vi "UHR-Fleezers Control (host) - 11.8.vi"() -> ()   [LabVIEW 2014] (continued)
                    tunnel: w545 -> [w549 w564]
                    tunnel: [w548 w563] -> w543
                    tunnel: w542 -> [_ w559]
                    frame False {
                      n310 = local read "Fish"() -> (w548:bool)
                      n311 = case shown="False" w548 {
                        tunnel: w549 -> [w550 _]
                        frame False {
                          n312 = property on="BD 1 Frequency 1 (MHz)" class="DigNum (strict)"("Val(Sgnl)"=w550) -> ()  [unwired: 2 in, 2 out]
                        }
                        frame True {
                        }
                      }
                    }
                    frame True {
                      w563 = FALSE ("Fish for Tether")
                      n313 = call <vilib>:"Beep.vi"() -> ()  [unwired: 3 in, 9 out]
                      n314 = Number To Decimal String(number=w559, width (-)=i16 1) -> (decimal integer string=w557:string)
                      n315 = Concatenate Strings("Formed tether in ", w557, " attempt(s)." ("string")) -> (w554:string)
                      n316 = local read "Messages"() -> (w561:string)
                      n317 = local write "Fish"(w563) -> ()
                      n318 = call "Update messages.vi"("Message to add"=w554, "Old message string"=w561) -> ("New message string"=w560:string)
                      n319 = local write "Messages"(w560) -> ()
                      n320 = Get Date/Time In Seconds() -> (seconds since 1Jan1904=→"Time tether formed":timestamp)
                      n321 = local read "Flow ON\nduring cal?"() -> (w551:bool)
                      n322 = property on="Sample Channel\nFlow" class="Bool (strict)"("Val(Sgnl)"=w551) -> (error out=w552:errorcluster)  [unwired: 2 in, 1 out]
                      n323 = case shown="\"8\"" "Then..." {
                        selector: "Then..." -> [_ w567 _ _]
                        tunnel: w564 -> [w566 _ _ _]
                        tunnel: w552 -> [_ _ _ _]
                        frame "1", Default {
                          n324 = property on="BD 1 Frequency 1 (MHz)" class="DigNum (strict)"("Val(Sgnl)"=w566) -> ()  [unwired: 2 in, 2 out]
                        }
                        frame "2", "3", "4", "5", "6" {
                          n325 = flat-sequence {
                            tunnel: w567 -> [w569]
                            frame #0 {
                              n326 = property on="Trap D (MHz)" class="DigNum (strict)"("Val(Sgnl)"="Move to D 1 (MHz)") -> ()  [unwired: 2 in, 2 out]
                            }
                            frame #1 {
                              n327 = case shown="\"2\", Default" w569 {
                                selector: w569 -> [w572 w582 _]
                                frame "3", "4" {
                                n328 = flat-sequence {
                                tunnel: w572 -> [w573]
                                tunnel: [w573] -> w570
                                tunnel: [w575] -> w571
                                tunnel: w570 -> [w575]
                                tunnel: w571 -> [w579]
                                frame #0 {
                                n329 = property on="Green Laser ON/Interlacing" class="Bool (strict)"("Val(Sgnl)"=TRUE ("Value (Signaling)")) -> ()  [unwired: 2 in, 2 out]
                                }
                                frame #1 {
                                n330 = Multiply(x="Wait Before Save (s)", y=u32 1000 ("x")) -> (x*y=w577:u32)
                                n331 = Wait (ms)(milliseconds to wait=w577) -> ()  [unwired: 1 out]
                                }
                                frame #2 {
                                n332 = property on="Start Saving" class="Bool (strict)"("Value"=TRUE ("Start Saving")) -> ()  [unwired: 2 in, 2 out]
                                n333 = case shown="\"4\"" w579 {
                                frame Default {
                                }
                                frame "4" {
                                n334 = property on="Fl. Triggered..." class="Bool (strict)"("Val(Sgnl)"=TRUE ("Value (Signaling)")) -> ()  [unwired: 2 in, 2 out]
                                }
                                }
                                }
                                }
                                }
                                frame "5", "6" {
                                n335 = stacked-sequence {
                                tunnel: w582 -> [_ _ _ _ _ _ w594]
                                frame #0 {
                                n336 = Replace Array Subset(array=u32[] [0] ("Index Values"), new element="Raster Set\nUpon Tether", index=0) -> (w583:u32[])
                                n337 = property on="Saved AOD Raster Scan Parameter Sets" class="Arr (strict)"("Index Values"=w583) -> ()  [unwired: 2 in, 2 out]
                                }
                                frame #1 {
                                n338 = Wait (ms)(milliseconds to wait=u32 500) -> ()  [unwired: 1 out]
                                }
                                frame #2 {
                                n339 = property on="Load parameters" class="Bool (strict)"("Val(Sgnl)"=TRUE ("Value (Signaling)")) -> ()  [unwired: 2 in, 2 out]
                                n340 = case shown="True" "Green ON during\nraster?" {
                                frame False {
                                }
                                frame True {
                                n341 = property on="Green Laser ON/Interlacing" class="Bool (strict)"("Val(Sgnl)"=TRUE ("Value (Signaling)")) -> ()  [unwired: 2 in, 2 out]
                                }
                                }
                                }
                                frame #3 {
                                n342 = Wait (ms)(milliseconds to wait=u32 500) -> ()  [unwired: 1 out]
                                }
                                frame #4 {
                                n343 = property on="Trap Raster Scan" class="Bool (strict)"("Val(Sgnl)"=TRUE ("Value (Signaling)")) -> ()  [unwired: 2 in, 2 out]
                                }
                                frame #5 {
                                n344 = Wait (ms)(milliseconds to wait=u32 2000) -> ()  [unwired: 1 out]
                                }
                                frame #6 {
                                n345 = flat-sequence {
                                tunnel: w594 -> [w601]
                                frame #0 {
                                n346 = while {
                                stop <- w597 stop-if-true
                                n347 = local read "Raster Scanning..."() -> (w596:bool)
                                n348 = local read "Saving..."() -> (w599:bool)
                                n349 = Wait (ms)(milliseconds to wait=u32 100) -> ()  [unwired: 1 out]
                                n350 = Not(x=w599) -> (.not. x?=w598:bool)
                                n351 = Not(x=w596) -> (.not. x?=w595:bool)
                                n352 = And(x=w598, y=w595) -> (x .and. y?=w597:bool)
                                }
                                }
                                frame #1 {
                                n353 = local read "Tether"() -> (w602:bool)
                                n354 = case shown="True" w602 {
                                tunnel: w601 -> [_ w604]
                                frame False {
                                n355 = property on="Fish" class="Bool (strict)"("Val(Sgnl)"="Fish again after \nraster break?") -> ()  [unwired: 2 in, 2 out]
                                }
                                frame True {
                                n356 = stacked-sequence {
                                tunnel: w604 -> [_ w608 _ _ _ _ _ _]
                                frame #0 {
                                n357 = property on="Trap D (MHz)" class="DigNum (strict)"("Val(Sgnl)"="Move to D 2 (MHz)") -> ()  [unwired: 2 in, 2 out]
                                n358 = case shown="True" "Flow ON after\ntether testing?" {
                                frame False {
                                }
                                frame True {
                                n359 = property on="Sample Channel\nFlow" class="Bool (strict)"("Val(Sgnl)"=TRUE ("Value (Signaling)")) -> ()  [unwired: 2 in, 2 out]
                                }
                                }
                                }
                                frame #1 {
                                n360 = flat-sequence {
                                tunnel: w608 -> [w609]
                                frame #0 {
                                n361 = case shown="\"6\"" w609 {
                                frame Default {
                                }
                                frame "6" {
                                n362 = flat-sequence {
                                frame #0 {
                                n363 = Wait (ms)(milliseconds to wait=u32 500) -> ()  [unwired: 1 out]
                                }
                                frame #1 {
                                n364 = property on="Green Laser ON/Interlacing" class="Bool (strict)"("Val(Sgnl)"=TRUE ("Green Laser ON/Interlacing")) -> ()  [unwired: 2 in, 2 out]
                                }
                                }
                                }
                                }
                                }
                                frame #1 {
                                n365 = case shown="True" "Save at end (5, 6)" {
                                selector: "Save at end (5, 6)" -> [_ w613]
                                frame False {
                                }
                                frame True {
                                n366 = flat-sequence {
                                tunnel: w613 -> [w615]
                                frame #0 {
                                n367 = Wait (ms)(milliseconds to wait=u32 500) -> ()  [unwired: 1 out]
                                }
                                frame #1 {
                                n368 = local write "Start Saving"(w615) -> ()
                                }
                                }
                                }
                                }
                                }
                                }
                                }
                                frame #2 {
                                n369 = local read "Bead Sep. Int. Time (s)"() -> (w618:dbl)
                                n370 = Multiply(x=w618, y=1000.0) -> (x*y=w617:dbl)
                                n371 = Wait (ms)(milliseconds to wait=w617) -> ()  [unwired: 1 out]
                                }
                                frame #3 {
                                n372 = property on="Remove Offset" class="Bool (strict)"("Val(Sgnl)"=TRUE ("Value (Signaling)")) -> ()  [unwired: 2 in, 2 out]
                                }
                                frame #4 {
                                n373 = property on="Read FX file" class="Bool (strict)"("Val(Sgnl)"=TRUE ("Value (Signaling)")) -> ()  [unwired: 2 in, 2 out]
                                }
                                frame #5 {
                                n374 = Wait (ms)(milliseconds to wait=u32 300) -> ()  [unwired: 1 out]
                                }
                                frame #6 {
                                n375 = local read "Bad fit error"() -> (w627:dbl)
                                n376 = local read "Fit offset"() -> (w630:dbl)
                                n377 = Greater Or Equal?(x=w627, y="Bad fit thresh") -> (x >= y?=→"Bad fit":bool)
                                n378 = Greater Or Equal?(x=w630, y="Fit offset thresh") -> (x >= y?=→"Multiple tether":bool)
                                n379 = local read "Hyst. error"() -> (w624:dbl)
                                n380 = Greater Or Equal?(x=w624, y="Hysteresis thresh") -> (x >= y?=→"Hysteresis":bool)
                                }
                                frame #7 {
                                w635 = 0
                                n381 = local read "Bad fit error"() -> (w637:dbl)
                                n382 = local read "Hyst. error"() -> (w636:dbl)
                                n383 = local read "Fit offset"() -> (w638:dbl)
                                n384 = local read "Multiple tether"() -> (w644:bool)
                                n385 = local read "Hysteresis"() -> (w642:bool)
                                n386 = local read "Bad fit"() -> (w643:bool)
                                n387 = Not(x=w642) -> (.not. x?=w634:bool)
                                n388 = Not(x=w643) -> (.not. x?=w640:bool)
                                n389 = Greater?(x=w638, y=w635) -> (0:w633:bool)
                                n390 = Greater?(x=w637, y=w635) -> (0:w632:bool)
                                n391 = Greater?(x=w636, y=w635) -> (0:w631:bool)
                                n392 = Not(x=w644) -> (.not. x?=w641:bool)
                                n393 = Compound Arithmetic op=AND(w641, w640, w634, w633, w632, w631) -> (w639:bool)
                                "Good tether" <- w639
                                n394 = case shown="True" w639 {
                                frame False {
                                }
                                frame True {
                                n395 = call <vilib>:"Beep.vi"("use system alert? (T)"=FALSE, "duration (msec)"=u32 200, "frequency (Hz)"=u32 2000) -> ()  [unwired: 9 in]
                                }
                                }
                                }
                                }
                                }
                                }
                                }
                                }
                                }
                                }
                                }
                                frame "2", Default {
                                }
                              }
                            }
                            frame #2 {
                              n396 = local read "Multiple tether"() -> (w650:bool)
                              n397 = And(x="Break multiple", y=w650) -> (x .and. y?=w648:bool)
                              n398 = case shown="True" w648 {
                                frame False {
                                }
                                frame True {
                                n399 = stacked-sequence {
                                frame #0 {
                                n400 = property on="Trap D (MHz)" class="DigNum (strict)"("Val(Sgnl)"="Trap D to \nbreak (MHz)") -> ()  [unwired: 2 in, 2 out]
                                }
                                frame #1 {
                                n401 = case shown="True" "Fish after\nmultiple break" {
                                frame False {
                                }
                                frame True {
                                n402 = while {
                                stop <- w655 stop-if-true
                                n403 = local read "Multiple tether"() -> (w657:bool)
                                n404 = local read "Fish"() -> (w654:bool)
                                n405 = local read "Stop All"() -> (w653:bool)
                                n406 = Wait (ms)(milliseconds to wait=u32 100) -> ()  [unwired: 1 out]
                                n407 = Not(x=w657) -> (.not. x?=w656:bool)
                                n408 = Compound Arithmetic op=OR(w653, w656, w654) -> (w655:bool)
                                }
                                }
                                }
                                }
                                frame #2 {
                                n409 = local read "Fish after\nmultiple break"() -> (w662:bool)
                                n410 = local read "Stage Moving"() -> (w661:bool)
                                n411 = Not(x=w661) -> (.not. x?=w659:bool)
                                n412 = And(x=w662, y=w659) -> (x .and. y?=w660:bool)
                                n413 = property on="Fish" class="Bool (strict)"("Val(Sgnl)"=w660) -> ()  [unwired: 2 in, 2 out]
                                }
                                }
                                }
                              }
                            }
                            frame #3 {
                              n414 = local read "Bad fit"() -> (w664:bool)
                              n415 = And(x="Break bad fit", y=w664) -> (x .and. y?=w663:bool)
                              n416 = case shown="True" w663 {
                                frame False {
                                }
                                frame True {
                                n417 = stacked-sequence {
                                frame #0 {
                                n418 = local read "Trap D to \nbreak (MHz)"() -> (w666:dbl)
                                n419 = property on="Trap D (MHz)" class="DigNum (strict)"("Val(Sgnl)"=w666) -> ()  [unwired: 2 in, 2 out]
                                }
                                frame #1 {
                                n420 = case shown="True" "Fish after\nbad fit break?" {
                                frame False {
                                }
                                frame True {
                                n421 = while {
                                stop <- w670 stop-if-true
                                n422 = local read "Stop All"() -> (w668:bool)
                                n423 = local read "Bad fit"() -> (w669:bool)
                                n424 = local read "Fish"() -> (w671:bool)
                                n425 = Not(x=w669) -> (.not. x?=w672:bool)
                                n426 = Wait (ms)(milliseconds to wait=u32 100) -> ()  [unwired: 1 out]
                                n427 = Compound Arithmetic op=OR(w668, w672, w671) -> (w670:bool)
                                }
                                }
                                }
                                }
                                frame #2 {
                                n428 = local read "Fish after\nbad fit break?"() -> (w674:bool)
                                n429 = local read "Stage Moving"() -> (w677:bool)
                                n430 = Not(x=w677) -> (.not. x?=w676:bool)
                                n431 = And(x=w674, y=w676) -> (x .and. y?=w675:bool)
                                n432 = property on="Fish" class="Bool (strict)"("Val(Sgnl)"=w675) -> ()  [unwired: 2 in, 2 out]
                                }
                                }
                                }
                              }
                            }
                            frame #4 {
                              n433 = local read "Hysteresis"() -> (w679:bool)
                              n434 = And(x="Break hyst", y=w679) -> (x .and. y?=w678:bool)
                              n435 = case shown="True" w678 {
                                frame False {
                                }
                                frame True {
                                n436 = stacked-sequence {
                                frame #0 {
                                n437 = local read "Trap D to \nbreak (MHz)"() -> (w681:dbl)
                                n438 = property on="Trap D (MHz)" class="DigNum (strict)"("Val(Sgnl)"=w681) -> ()  [unwired: 2 in, 2 out]
                                }
                                frame #1 {
                                n439 = case shown="True" "Fish ater hyst?" {
                                frame False {
                                }
                                frame True {
                                n440 = while {
                                stop <- w687 stop-if-true
                                n441 = local read "Hysteresis"() -> (w686:bool)
                                n442 = local read "Stop All"() -> (w683:bool)
                                n443 = local read "Fish"() -> (w684:bool)
                                n444 = Wait (ms)(milliseconds to wait=u32 100) -> ()  [unwired: 1 out]
                                n445 = Not(x=w686) -> (.not. x?=w685:bool)
                                n446 = Compound Arithmetic op=OR(w683, w685, w684) -> (w687:bool)
                                }
                                }
                                }
                                }
                                frame #2 {
                                n447 = local read "Fish ater hyst?"() -> (w692:bool)
                                n448 = local read "Stage Moving"() -> (w691:bool)
                                n449 = Not(x=w691) -> (.not. x?=w690:bool)
                                n450 = And(x=w692, y=w690) -> (x .and. y?=w689:bool)
                                n451 = property on="Fish" class="Bool (strict)"("Val(Sgnl)"=w689) -> ()  [unwired: 2 in, 2 out]
                                }
                                }
                                }
                              }
                            }
                            frame #5 {
                              n452 = local read "Good tether"() -> (w693:bool)
                              n453 = case shown="True" w693 {
                                frame False {
                                }
                                frame True {
                                n454 = case shown="\"1\"" "If good, then:" {
                                frame "0", Default {
                                }
                                frame "1" {
                                n455 = property on="Force FB Script" class="Bool (strict)"("Val(Sgnl)"=TRUE ("Value (Signaling)")) -> ()  [unwired: 2 in, 2 out]
                                }
                                }
                                }
                              }
                            }
                          }
                        }
                        frame "7" {
                          n456 = property on="Force FB Script" class="Bool (strict)"("Val(Sgnl)"=TRUE ("Value (Signaling)")) -> ()  [unwired: 2 in, 2 out]
                        }
                        frame "8" {
                          n457 = property on="Fixed Traps Script" class="Bool (strict)"("Val(Sgnl)"=TRUE ("Value (Signaling)")) -> ()  [unwired: 2 in, 2 out]
                        }
                      }
                      "Tether" <- "Tether Alarm?"
                    }
                  }
                }
                frame #2 {
                  n458 = local read "Oscillate Set 1"() -> (w703:bool)
                  n459 = local read "Stop All"() -> (w701:bool)
                  n460 = Or(x=w703, y=w698) -> (x .or. y?=w700:bool)
                  n461 = Not(x=w700) -> (.not. x?=w702:bool)
                  n462 = Compound Arithmetic op=OR(w701, w702) -> (w699:bool)
                }
              }
              n463 = node-c288() -> ()  [unwired: 2 out]
            }
            n464 = node-c288(w457) -> ()  [unwired: 1 out]
          }
        }
      }
      event "Fl. Triggered...": Value Change {
        n465 = event-data() -> ()  [unwired: 7 out]
        n466 = case shown="True" "Fl. Triggered..." {
          frame False {
          }
          frame True {
            n467 = node-c288() -> (w714:T21)  [unwired: 4 out]
            n468 = timed-loop {
              timing: w714 -> [_]
              timing-out: [_] -> w713
              tunnel: "Action" -> [w722]
              shift-right: [w719] -> _
              shift-left: u8 255 -> [w721]
              shift-right: [w716] -> _
              shift-left: 255 -> [w718]
              stop <- w715 stop-if-true
              # "Reset confocal spot"
              n469 = node-c288() -> ()  [unwired: 2 out]
              n470 = flat-sequence {
                tunnel: w722 -> [w742]
                tunnel: w721 -> [w741]
                tunnel: [w740] -> w720
                tunnel: w718 -> [w727]
                tunnel: [w726] -> w717
                tunnel: [w1126] -> w715
                tunnel: w720 -> [w1125]
                tunnel: [w1125] -> w719
                tunnel: [w1124] -> w716
                tunnel: w717 -> [w1124]
                frame #0 {
                  n471 = local read "Delta Fl. 2"() -> (w739:dbl)
                  n472 = local read "Delta Fl. 1"() -> (w734:dbl)
                  n473 = Multiply(x="Fl. D Thresh. (kHz)", y=1000.0) -> (x*y=w729:dbl)
                  n474 = Select(t=w734, s="APD to Watch", f=w739) -> (s? t:f=w730:dbl)
                  n475 = Greater?(x=w730, y=w729) -> (0:w735:bool)
                  n476 = Or(x="Force Yank", y=w735) -> (x .or. y?=w733:bool)
                  n477 = And(x=w733, y="Yank when?") -> (x .and. y?=w731:bool)
                  n478 = case shown="False" w731 {
                    tunnel: w742 -> [w745 w948]
                    tunnel: w741 -> [w747 w944]
                    tunnel: [w747 w942] -> w740
                    tunnel: w730 -> [w753 _]
                    tunnel: w729 -> [w752 _]
                    tunnel: "Force Yank" -> [w750 _]
                    tunnel: w727 -> [w749 w941]
                    tunnel: [w748 w941] -> w726
                    frame False {
                      n479 = Negate(x=w752) -> (-x=w744:dbl)
                      n480 = local write "Fl. High"(TRUE ("Fl. High")) -> ()
                      n481 = Less?(x=w753, y=w744) -> (x < y?=w751:bool)
                      n482 = Or(x=w750, y=w751) -> (x .or. y?=w746:bool)
                      n483 = case shown="True" w746 {
                        tunnel: w749 -> [w754 w764]
                        tunnel: [w754 w763] -> w748
                        tunnel: w745 -> [_ w762]
                        frame False {
                        }
                        frame True {
                          n484 = flat-sequence {
                            tunnel: w764 -> [w770]
                            tunnel: w762 -> [w767]
                            tunnel: [w769] -> w761
                            tunnel: [w768] -> w760
                            tunnel: [w767] -> w759
                            tunnel: w758 -> [w766]
                            tunnel: [w766] -> w757
                            tunnel: w756 -> [w765]
                            tunnel: [w765] -> w755
                            tunnel: [w842] -> w763
                            tunnel: w761 -> [w842]
                            tunnel: w760 -> [w841]
                            tunnel: w759 -> [w840]
                            tunnel: w757 -> [w839]
                            tunnel: w755 -> [w838]
                            frame #0 {
                              n485 = call <vilib>:"Beep.vi"() -> ()  [unwired: 12 in]
                              n486 = local write "Waiting"(FALSE ("Waiting")) -> ()
                              n487 = Increment(x=w770) -> (x+1=w769:i32)
                              n488 = case shown="\"Yank\"" w767 {
                                tunnel: w769 -> [_ w775 _]
                                frame "Alarm", Default {
                                }
                                frame "Yank" {
                                n489 = flat-sequence {
                                tunnel: w775 -> [w778]
                                tunnel: [w777] -> w774
                                tunnel: [w776] -> w773
                                tunnel: w774 -> [w788]
                                tunnel: w773 -> [w789]
                                frame #0 {
                                n490 = local read "Yank Delay (s)"() -> (w781:dbl)
                                n491 = local read "N Array El"() -> (w776:u8)
                                n492 = Quotient & Remainder(x=w778, y=w776) -> (x-y*floor(x/y)=w777:i32)  [unwired: 1 out]
                                n493 = Multiply(x=w781, y=1000.0) -> (x*y=w779:dbl)
                                n494 = Wait (ms)(milliseconds to wait=w779) -> ()  [unwired: 1 out]
                                }
                                frame #1 {
                                n495 = local read "Yank to which?"() -> (w783:bool)
                                n496 = local read "Random Choice"() -> (w793:bool)
                                n497 = local read "Yank to Trap D (MHz)"() -> (w786:dbl[])
                                n498 = local read "Yank to SP"() -> (w787:dbl[])
                                n499 = Random Number (0-1)() -> (number: 0 to 1=w792:dbl)
                                n500 = Multiply(x=w789, y=w792) -> (x*y=w791:dbl)
                                n501 = Round Toward -Infinity(1:w791) -> (0:w790:dbl)
                                n502 = Select(t=w790, s=w793, f=w788) -> (s? t:f=w784:dbl)
                                n503 = Select(t=w786, s=w783, f=w787) -> (s? t:f=w785:dbl[])
                                n504 = Index Array(array=w785, index=w784) -> (element=w782:dbl)
                                n505 = case shown="False" w783 {
                                tunnel: w782 -> [w794 w822]
                                frame False {
                                n506 = flat-sequence {
                                tunnel: w794 -> [w795]
                                frame #0 {
                                n507 = property on="Trap Pos FB SP" class="DigNum (strict)"("Val(Sgnl)"=w795) -> ()  [unwired: 2 in, 2 out]
                                }
                                frame #1 {
                                n508 = Wait (ms)(milliseconds to wait=u32 700) -> ()  [unwired: 1 out]
                                }
                                frame #2 {
                                n509 = local read "Action (%)"() -> (w800:dbl)
                                n510 = Absolute Value(x=w800) -> (abs(x)=w799:dbl)
                                n511 = Greater?(x=w799, y=70.0) -> (0:w797:bool)
                                n512 = property on="Remove Action Offset" class="Bool (strict)"("Val(Sgnl)"=w797) -> ()  [unwired: 2 in, 2 out]
                                }
                                frame #3 {
                                n513 = for {
                                N: 4 -> [_]
                                n514 = flat-sequence {
                                frame #0 {
                                n515 = Wait (ms)(milliseconds to wait=u32 500) -> ()  [unwired: 1 out]
                                }
                                frame #1 {
                                n516 = local read "Action (%)"() -> (w806:dbl)
                                n517 = Absolute Value(x=w806) -> (abs(x)=w805:dbl)
                                n518 = Greater?(x=w805, y=70.0) -> (0:w803:bool)
                                n519 = property on="Remove Action Offset" class="Bool (strict)"("Val(Sgnl)"=w803) -> ()  [unwired: 2 in, 2 out]
                                }
                                }
                                }
                                }
                                frame #4 {
                                n520 = Wait (ms)(milliseconds to wait=u32 500) -> ()  [unwired: 1 out]
                                }
                                frame #5 {
                                n521 = local read "Mean"() -> (w814:dbl)
                                n522 = Greater?(x=w814, y=11.0) -> (0:w808:bool)
                                n523 = Not(x=w808) -> (.not. x?=w809:bool)
                                n524 = And(x=w809, y="Shift confocal") -> (x .and. y?=w811:bool)
                                n525 = And(x=w808, y="Shift confocal") -> (x .and. y?=w812:bool)
                                n526 = case shown="True" w812 {
                                frame False {
                                }
                                frame True {
                                n527 = local read "Confocal Y 2 (V)"() -> (w818:dbl)
                                n528 = local read "Confocal X 2 (V)"() -> (w817:dbl)
                                n529 = property on="AO1" class="Slide (strict)"("Val(Sgnl)"=w818) -> ()  [unwired: 2 in, 2 out]
                                n530 = property on="AO2" class="Slide (strict)"("Val(Sgnl)"=w817) -> ()  [unwired: 2 in, 2 out]
                                }
                                }
                                n531 = case shown="True" w811 {
                                frame False {
                                }
                                frame True {
                                n532 = local read "Confocal Y 1 (V)"() -> (w816:dbl)
                                n533 = local read "Confocal X 1 (V)"() -> (w815:dbl)
                                n534 = property on="AO1" class="Slide (strict)"("Val(Sgnl)"=w816) -> ()  [unwired: 2 in, 2 out]
                                n535 = property on="AO2" class="Slide (strict)"("Val(Sgnl)"=w815) -> ()  [unwired: 2 in, 2 out]
                                }
                                }
                                }
                                frame #6 {
                                n536 = Wait (ms)(milliseconds to wait=u32 1500) -> ()  [unwired: 1 out]
                                }
                                frame #7 {
                                n537 = property on="Rem fb disp offset" class="Bool (strict)"("Val(Sgnl)"=TRUE ("Value (Signaling)")) -> ()  [unwired: 2 in, 2 out]
                                n538 = property on="Remove Offset" class="Bool (strict)"("Val(Sgnl)"=TRUE ("Value (Signaling)")) -> ()  [unwired: 2 in, 2 out]
                                }
                                }
                                }
                                frame True {
                                n539 = flat-sequence {
                                tunnel: w822 -> [w823]
                                frame #0 {
                                n540 = property on="Trap D (MHz)" class="DigNum (strict)"("Val(Sgnl)"=w823) -> ()  [unwired: 2 in, 2 out]
                                }
                                frame #1 {
                                n541 = Wait (ms)(milliseconds to wait=u32 500) -> ()  [unwired: 1 out]
                                }
                                frame #2 {
                                n542 = local read "Shift confocal"() -> (w829:bool)
                                n543 = local read "Mean"() -> (w831:dbl)
                                n544 = Greater?(x=w831, y=11.0) -> (0:w828:bool)
                                n545 = Not(x=w828) -> (.not. x?=w827:bool)
                                n546 = And(x=w827, y=w829) -> (x .and. y?=w825:bool)
                                n547 = And(x=w828, y=w829) -> (x .and. y?=w826:bool)
                                n548 = case shown="True" w826 {
                                frame False {
                                }
                                frame True {
                                n549 = local read "Confocal Y 2 (V)"() -> (w835:dbl)
                                n550 = local read "Confocal X 2 (V)"() -> (w834:dbl)
                                n551 = property on="AO2" class="Slide (strict)"("Val(Sgnl)"=w834) -> ()  [unwired: 2 in, 2 out]
                                n552 = property on="AO1" class="Slide (strict)"("Val(Sgnl)"=w835) -> ()  [unwired: 2 in, 2 out]
                                }
                                }
                                n553 = case shown="True" w825 {
                                frame False {
                                }
                                frame True {
                                n554 = local read "Confocal X 1 (V)"() -> (w832:dbl)
                                n555 = local read "Confocal Y 1 (V)"() -> (w833:dbl)
                                n556 = property on="AO2" class="Slide (strict)"("Val(Sgnl)"=w832) -> ()  [unwired: 2 in, 2 out]
                                n557 = property on="AO1" class="Slide (strict)"("Val(Sgnl)"=w833) -> ()  [unwired: 2 in, 2 out]
                                }
                                }
                                }
                                }
                                }
                                }
                                }
                                }
                                }
                                frame "Image" {
                                n558 = property on="Confocal\nImage" class="Bool (strict)"("Val(Sgnl)"=TRUE ("Value (Signaling)")) -> ()  [unwired: 2 in, 2 out]
                                }
                              }
                              n559 = local write "Fl. High"(FALSE ("Fl. High")) -> ()
                              n560 = local read "Time (s)"() -> (w768:dbl)
                            }
                            frame #1 {
                              n561 = case shown="True" "Auto F Reset" {
                                tunnel: w841 -> [_ w846]
                                tunnel: w840 -> [_ w845]
                                tunnel: w839 -> [_ w844]
                                tunnel: w838 -> [_ w843]
                                frame False {
                                }
                                frame True {
                                n562 = node-c288() -> (w848:T21)  [unwired: 4 in]
                                n563 = timed-loop {
                                timing: w848 -> [_]
                                timing-out: [_] -> w847
                                tunnel: w846 -> [w853]
                                tunnel: w845 -> [w852]
                                tunnel: w844 -> [w851]
                                tunnel: w843 -> [w850]
                                stop <- w849 stop-if-true
                                n564 = node-c288() -> ()  [unwired: 1 in, 1 out]
                                n565 = local read "APD to Watch"() -> (w863:bool)
                                n566 = local read "Fl. D Thresh. (kHz)"() -> (w862:dbl)
                                n567 = local read "Delta Fl. 1"() -> (w864:dbl)
                                n568 = local read "Delta Fl. 2"() -> (w865:dbl)
                                n569 = local read "Fl. Triggered..."() -> (w856:bool)
                                n570 = local read "Stop All"() -> (w857:bool)
                                n571 = local read "Reset Force"() -> (w855:bool)
                                n572 = Multiply(x=w862, y=1000.0) -> (x*y=w860:dbl)
                                n573 = Not(x=w856) -> (.not. x?=w854:bool)
                                n574 = Select(t=w864, s=w863, f=w865) -> (s? t:f=w859:dbl)
                                n575 = Greater?(x=w859, y=w860) -> (0:w858:bool)
                                n576 = Compound Arithmetic op=OR(w858, w857, w854, w855) -> (w849:bool)
                                n577 = case shown="True" w849 {
                                tunnel: w853 -> [_ w869]
                                tunnel: w852 -> [_ w873]
                                tunnel: w851 -> [_ w872]
                                tunnel: w850 -> [_ w871]
                                frame False {
                                }
                                frame True {
                                n578 = case shown="\"Yank\"" w873 {
                                tunnel: w872 -> [_ w883]
                                tunnel: w871 -> [_ w881]
                                frame "Image", Default {
                                }
                                frame "Yank" {
                                n579 = flat-sequence {
                                tunnel: [w886] -> w884
                                tunnel: w883 -> [w886]
                                tunnel: [w885] -> w882
                                tunnel: w881 -> [w885]
                                tunnel: w884 -> [w892]
                                tunnel: w882 -> [w890]
                                frame #0 {
                                n580 = local read "Yank Delay (s)"() -> (w889:dbl)
                                n581 = Multiply(x=w889, y=1000.0) -> (x*y=w887:dbl)
                                n582 = Wait (ms)(milliseconds to wait=w887) -> ()  [unwired: 1 out]
                                }
                                frame #1 {
                                n583 = local read "Yank to which?"() -> (w891:bool)
                                n584 = case shown="False" w891 {
                                tunnel: w892 -> [_ w921]
                                tunnel: w890 -> [w893 _]
                                frame False {
                                n585 = flat-sequence {
                                tunnel: w893 -> [w894]
                                frame #0 {
                                n586 = property on="Trap Pos FB SP" class="DigNum (strict)"("Val(Sgnl)"=w894) -> ()  [unwired: 2 in, 2 out]
                                }
                                frame #1 {
                                n587 = Wait (ms)(milliseconds to wait=u32 700) -> ()  [unwired: 1 out]
                                }
                                frame #2 {
                                n588 = local read "Action (%)"() -> (w899:dbl)
                                n589 = Absolute Value(x=w899) -> (abs(x)=w898:dbl)
                                n590 = Greater?(x=w898, y=70.0) -> (0:w896:bool)
                                n591 = property on="Remove Action Offset" class="Bool (strict)"("Val(Sgnl)"=w896) -> ()  [unwired: 2 in, 2 out]
                                }
                                frame #3 {
                                n592 = for {
                                N: 4 -> [_]
                                n593 = flat-sequence {
                                frame #0 {
                                n594 = Wait (ms)(milliseconds to wait=u32 500) -> ()  [unwired: 1 out]
                                }
                                frame #1 {
                                n595 = local read "Action (%)"() -> (w905:dbl)
                                n596 = Absolute Value(x=w905) -> (abs(x)=w904:dbl)
                                n597 = Greater?(x=w904, y=70.0) -> (0:w902:bool)
                                n598 = property on="Remove Action Offset" class="Bool (strict)"("Val(Sgnl)"=w902) -> ()  [unwired: 2 in, 2 out]
                                }
                                }
                                }
                                }
                                frame #4 {
                                n599 = Wait (ms)(milliseconds to wait=u32 500) -> ()  [unwired: 1 out]
                                }
                                frame #5 {
                                n600 = local read "Shift confocal"() -> (w910:bool)
                                n601 = local read "Mean"() -> (w913:dbl)
                                n602 = Greater?(x=w913, y=11.0) -> (0:w909:bool)
                                n603 = Not(x=w909) -> (.not. x?=w908:bool)
                                n604 = And(x=w909, y=w910) -> (x .and. y?=w911:bool)
                                n605 = And(x=w908, y=w910) -> (x .and. y?=w907:bool)
                                n606 = case shown="True" w911 {
                                frame False {
                                }
                                frame True {
                                n607 = local read "Confocal X 2 (V)"() -> (w916:dbl)
                                n608 = local read "Confocal Y 2 (V)"() -> (w917:dbl)
                                n609 = property on="AO2" class="Slide (strict)"("Val(Sgnl)"=w916) -> ()  [unwired: 2 in, 2 out]
                                n610 = property on="AO1" class="Slide (strict)"("Val(Sgnl)"=w917) -> ()  [unwired: 2 in, 2 out]
                                }
                                }
                                n611 = case shown="True" w907 {
                                frame False {
                                }
                                frame True {
                                n612 = local read "Confocal Y 1 (V)"() -> (w915:dbl)
                                n613 = local read "Confocal X 1 (V)"() -> (w914:dbl)
                                n614 = property on="AO1" class="Slide (strict)"("Val(Sgnl)"=w915) -> ()  [unwired: 2 in, 2 out]
                                n615 = property on="AO2" class="Slide (strict)"("Val(Sgnl)"=w914) -> ()  [unwired: 2 in, 2 out]
                                }
                                }
                                }
                                frame #6 {
                                n616 = Wait (ms)(milliseconds to wait=u32 1500) -> ()  [unwired: 1 out]
                                }
                                frame #7 {
                                n617 = property on="Remove Offset" class="Bool (strict)"("Val(Sgnl)"=TRUE ("Value (Signaling)")) -> ()  [unwired: 2 in, 2 out]
                                n618 = property on="Rem fb disp offset" class="Bool (strict)"("Val(Sgnl)"=TRUE ("Value (Signaling)")) -> ()  [unwired: 2 in, 2 out]
                                }
                                }
                                }
                                frame True {
                                n619 = flat-sequence {
                                tunnel: w921 -> [w922]
                                frame #0 {
                                n620 = property on="Trap D (MHz)" class="DigNum (strict)"("Val(Sgnl)"=w922) -> ()  [unwired: 2 in, 2 out]
                                }
                                frame #1 {
                                n621 = Wait (ms)(milliseconds to wait=u32 500) -> ()  [unwired: 1 out]
                                }
                                frame #2 {
                                n622 = local read "Shift confocal"() -> (w928:bool)
                                n623 = local read "Mean"() -> (w929:dbl)
                                n624 = Greater?(x=w929, y=11.0) -> (0:w927:bool)
                                n625 = And(x=w927, y=w928) -> (x .and. y?=w925:bool)
                                n626 = Not(x=w927) -> (.not. x?=w926:bool)
                                n627 = And(x=w926, y=w928) -> (x .and. y?=w924:bool)
                                n628 = case shown="True" w925 {
                                frame False {
                                }
                                frame True {
                                n629 = local read "Confocal Y 2 (V)"() -> (w934:dbl)
                                n630 = local read "Confocal X 2 (V)"() -> (w933:dbl)
                                n631 = property on="AO1" class="Slide (strict)"("Val(Sgnl)"=w934) -> ()  [unwired: 2 in, 2 out]
                                n632 = property on="AO2" class="Slide (strict)"("Val(Sgnl)"=w933) -> ()  [unwired: 2 in, 2 out]
                                }
                                }
                                n633 = case shown="True" w924 {
                                frame False {
                                }
                                frame True {
                                n634 = local read "Confocal Y 1 (V)"() -> (w932:dbl)
                                n635 = local read "Confocal X 1 (V)"() -> (w931:dbl)
                                n636 = property on="AO2" class="Slide (strict)"("Val(Sgnl)"=w931) -> ()  [unwired: 2 in, 2 out]
                                n637 = property on="AO1" class="Slide (strict)"("Val(Sgnl)"=w932) -> ()  [unwired: 2 in, 2 out]
                                }
                                }
                                }
                                }
                                }
                                }
                                }
                                }
                                }
                                }
                                n638 = local read "Time (s)"() -> (w868:dbl)
                                n639 = Subtract(x=w869, y=w868) -> (x-y=w880:dbl)
                                n640 = Number To Decimal String(number=w880, width (-)=i16 0) -> (decimal integer string=w878:string)
                                n641 = Concatenate Strings(w878, " s fluorescence event") -> (w875:string)
                                n642 = local read "Messages"() -> (w876:string)
                                n643 = local write "Duration (s)"(w880) -> ()
                                n644 = call "Update messages.vi"("Message to add"=w875, "Old message string"=w876) -> ("New message string"=w874:string)
                                n645 = local write "Messages"(w874) -> ()
                                n646 = call <vilib>:"Beep.vi"() -> ()  [unwired: 12 in]
                                n647 = local write "Reset Force"(FALSE ("Force Reset")) -> ()
                                n648 = local write "Fl. High"(TRUE ("Fl. High")) -> ()
                                n649 = local write "Waiting"(TRUE ("Waiting")) -> ()
                                }
                                }
                                n650 = node-c288() -> ()  [unwired: 1 in, 1 out]
                                }
                                n651 = node-c288(w847) -> ()  [unwired: 1 out]
                                }
                              }
                            }
                          }
                          n652 = local read "Trap Pos FB SP"() -> (w756:fxp<+/-,16,1>)
                          n653 = local read "Trap D (MHz)"() -> (w758:dbl)
                        }
                      }
                    }
                    frame True {
                      n654 = flat-sequence {
                        tunnel: w945 -> [w955]
                        tunnel: [w955] -> w949
                        tunnel: w948 -> [w954]
                        tunnel: [w954] -> w947
                        tunnel: [w953] -> w946
                        tunnel: w944 -> [w952]
                        tunnel: [w951] -> w943
                        tunnel: w940 -> [w950]
                        tunnel: [w950] -> w939
                        tunnel: w949 -> [w1027]
                        tunnel: w947 -> [w1026]
                        tunnel: w946 -> [w1025]
                        tunnel: w943 -> [w1024]
                        tunnel: w939 -> [w1023]
                        tunnel: [w1024] -> w942
                        frame #0 {
                          n655 = call <vilib>:"Beep.vi"() -> ()  [unwired: 3 in, 9 out]
                          n656 = local write "Waiting"(FALSE ("Waiting")) -> ()
                          n657 = Increment(x=w952) -> (x+1=w951:u8)
                          n658 = case shown="\"Image\"" w954 {
                            tunnel: w951 -> [_ _ w961 _]
                            frame "Image" {
                              n659 = property on="Confocal\nImage" class="Bool (strict)"("Val(Sgnl)"=TRUE ("Value (Signaling)")) -> ()  [unwired: 2 in, 2 out]
                            }
                            frame "Alarm", Default {
                            }
                            frame "Yank" {
                              n660 = flat-sequence {
                                tunnel: w961 -> [w964]
                                tunnel: [w963] -> w960
                                tunnel: ["N Array El"] -> w959
                                tunnel: w960 -> [w978]
                                tunnel: w959 -> [w974]
                                frame #0 {
                                n661 = Multiply(x="Yank Delay (s)", y=1000.0) -> (x*y=w967:dbl)
                                n662 = Quotient & Remainder(x=w964, y="N Array El") -> (x-y*floor(x/y)=w963:u8)  [unwired: 1 out]
                                n663 = Wait (ms)(milliseconds to wait=w967) -> ()  [unwired: 1 out]
                                }
                                frame #1 {
                                n664 = Random Number (0-1)() -> (number: 0 to 1=w975:dbl)
                                n665 = Multiply(x=w974, y=w975) -> (x*y=w973:dbl)
                                n666 = Round Toward -Infinity(1:w973) -> (0:w972:dbl)
                                n667 = Select(t=w972, s="Random Choice", f=w978) -> (s? t:f=w976:dbl)
                                n668 = Select(t="Yank to Trap D (MHz)", s="Yank to which?", f="Yank to SP") -> (s? t:f=w969:dbl[])
                                n669 = Index Array(array=w969, index=w976) -> (element=w979:dbl)
                                n670 = case shown="False" "Yank to which?" {
                                tunnel: w979 -> [w980 w1007]
                                frame False {
                                n671 = flat-sequence {
